vi "OtherSideFrom.vi"(8 "error in (no error)":errorcluster, 10 "Room* in":refnum<data-value>, 11 "Door in":refnum<class "Door.lvclass">) -> (0 "error out":errorcluster, 2 "Room* out":refnum<data-value>, 3 "Door out":refnum<class "Door.lvclass">)   [LabVIEW 2016, in "Door.lvclass"]
uses:
  Door.lvclass
  Room/Room.lvclass
  Door.lvclass/Door.ctl
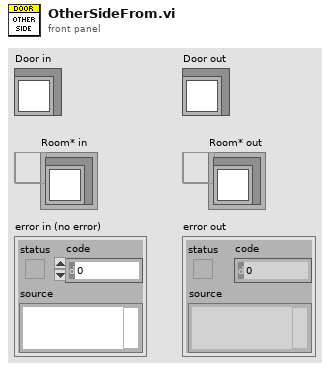
[diagram p1: front panel]
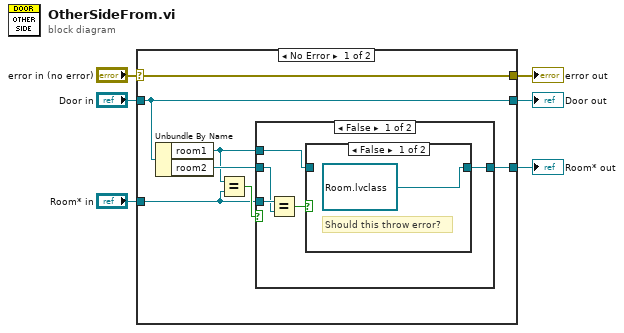
[diagram p0: block diagram]
diagram:
  n1 = case shown="No Error" "error in (no error)" {
    selector: "error in (no error)" -> [w13 w23]
    tunnel: [w13 w23] -> w5
    tunnel: [w12 w22] -> w3
    tunnel: "Door in" -> [w12 w22]
    tunnel: "Room* in" -> [w8 _]
    tunnel: [w10 _] -> w1
    frame No Error {
      n2 = Unbundle By Name(w12) -> ("room1"=w7:refnum<data-value>, "room2"=w9:refnum<data-value>)
      n3 = Equal?(x=w7, y=w8) -> (x = y?=w11:bool)
      n4 = case shown="False" w11 {
        tunnel: [w15 w21] -> w10
        tunnel: w9 -> [w17 w21]
        tunnel: w8 -> [w18 _]
        tunnel: w7 -> [w14 _]
        frame False {
          n5 = Equal?(x=w18, y=w17) -> (x = y?=w16:bool)
          n6 = case shown="False" w16 {
            tunnel: [refnum<data-value> refnum ("room1") w20] -> w15
            tunnel: w14 -> [_ w20]
            frame False {
              # "Should this throw error?"
            }
            frame True {
            }
          }
        }
        frame True {
        }
      }
    }
    frame Error {
    }
  }
  "error out" <- w5
  "Door out" <- w3
  "Room* out" <- w1
